vi "HTTPMethod_Synchronous_Simple.vi"(0 "LabVIEWHTTPClient_NET in":refnum<class "HttpClient_NET.lvclass">, 1 "input file":path, 2 "Method":T2, 3 "output file":path, 5 "URL":string, 7 "buffer":string, 9 "request headers":cluster{"header":string, "value":string}[](array[cluster]), 11 "error in (no error)":errorcluster, 12 "Timeout_ms (10000)":i32=10000) -> (4 "LabVIEWHTTPClient_NET out":refnum<class "HttpClient_NET.lvclass">, 6 "Headers":T1, 8 "Response":string, 10 "StatusCode":i32(ring)=100 items=["Continue"=100, "SwitchingProtocols"=101, "OK"=200, "Created"=201, "Accepted"=202, "NonAuthoritativeInformation"=203, "NoContent"=204, "ResetContent"=205, "PartialContent"=206, "MultipleChoices, Ambiguous"=300, "MovedPermanently, Moved"=301, "Found, Redirect"=302, "SeeOther, RedirectMethod"=303, "NotModified"=304, "UseProxy"=305, "Unused"=306, "TemporaryRedirect, RedirectKeepVerb"=307, "BadRequest"=400, "Unauthorized"=401, "PaymentRequired"=402, "Forbidden"=403, "NotFound"=404, "MethodNotAllowed"=405, "NotAcceptable"=406, "ProxyAuthenticationRequired"=407, "RequestTimeout"=408, "Conflict"=409, "Gone"=410, "LengthRequired"=411, "PreconditionFailed"=412, "RequestEntityTooLarge"=413, "RequestUriTooLong"=414, "UnsupportedMediaType"=415, "RequestedRangeNotSatisfiable"=416, "ExpectationFailed"=417, "UpgradeRequired"=426, "InternalServerError"=500, "NotImplemented"=501, "BadGateway"=502, "ServiceUnavailable"=503, "GatewayTimeout"=504, "HttpVersionNotSupported"=505], 13 "ReasonPhrase":string, 14 "Timeout":bool, 15 "error out":errorcluster)   [LabVIEW 2018, in "HttpClient_NET.lvlib" / "HttpClient_NET.lvclass"]
doc: "<b> </b> <b> </b>\nHttpClient_NET\nJustin Young - Viviota\nCopyright (c) 2021\nLicense: BSD"
uses:
  HttpClient_NET.lvclass
  Types/method_enum.ctl
  Types/ResponseHeaders_Cluster.ctl
  HttpHeaders_response/HttpHeaders_Response.lvclass
  HttpHeaders_content/HttpHeaders_Content.lvclass
  HttpResponseMessage/HttpResponseMessage.lvclass
  HttpRequestMessage/HttpRequestMessage.lvclass
  HttpClient_NET.lvlib
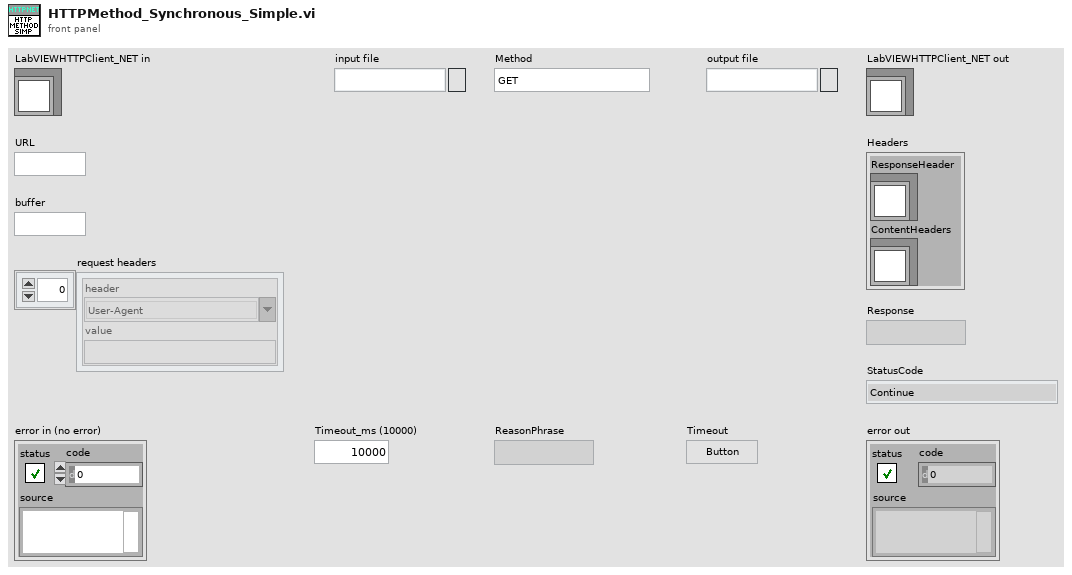
[diagram p1: front panel]
types:
  T1 = typedef "HttpClient_NET.lvlib/ResponseHeaders_Cluster.ctl" = cluster{"ResponseHeader":refnum<class "HttpHeaders_Response.lvclass">, "ContentHeaders":refnum<class "HttpHeaders_Content.lvclass">}
  T2 = typedef "HttpClient_NET.lvlib/method_enum.ctl" = enum16{"GET", "PUT", "POST", "DELETE", "HEAD", "TRACE", "SEND"}
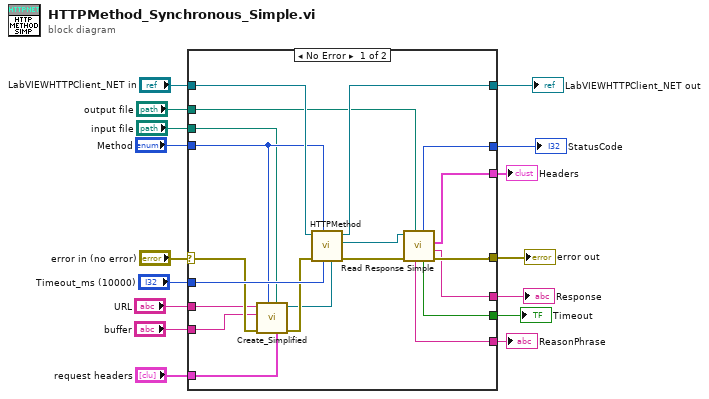
[diagram p0: block diagram]
diagram:
  n1 = case shown="No Error" "error in (no error)" {
    selector: "error in (no error)" -> [w25 w38]
    tunnel: [w32 w38] -> w15
    tunnel: [w34 w37] -> w13
    tunnel: "LabVIEWHTTPClient_NET in" -> [w35 w37]
    tunnel: "Method" -> [w22 _]
    tunnel: "Timeout_ms (10000)" -> [w36 _]
    tunnel: "URL" -> [w21 _]
    tunnel: "output file" -> [w30 _]
    tunnel: [w29 _] -> w8
    tunnel: [w28 _] -> w7
    tunnel: [w27 _] -> w3
    tunnel: [w26 _] -> w2
    tunnel: "input file" -> [w20 _]
    tunnel: "buffer" -> [w19 _]
    tunnel: "request headers" -> [w18 _]
    tunnel: [w17 _] -> w1
    frame No Error {
      n2 = call "Create_Simplified.vi"("request headers"=w18, "input file"=w20, "Method [GET]"=w22, "error in (no error)"=w25, "buffer"=w19, "Address"=w21) -> ("error out"=w24:errorcluster, "HttpRequestMessage out"=w23:refnum<class "HttpRequestMessage.lvclass">)  [unwired: 3 in, 1 out]
      n3 = call "HTTPMethod.vi"("HttpRequestMessage"=w23, "Timeout_ms (10000)"=w36, "Method"=w22, "error in (no error)"=w24, "LabVIEWHTTPClient_NET in"=w35) -> ("error out"=w33:errorcluster, "HttpResponseMessage out"=w31:refnum<class "HttpResponseMessage.lvclass">, "LabVIEWHTTPClient_NET out"=w34:refnum<class "HttpClient_NET.lvclass">)  [unwired: 4 in]
      n4 = call "Read Response Simple.vi"("output file"=w30, "error in (no error)"=w33, "HttpResponseMessage in"=w31) -> ("error out"=w32:errorcluster, "Response"=w28:string, "Headers"=w26:T1, "Timeout"=w29:bool, "StatusCode"=w27:i32, "ReasonPhrase"=w17:string)  [unwired: 3 in]
    }
    frame Error {
    }
  }
  "error out" <- w15
  "LabVIEWHTTPClient_NET out" <- w13
  "Timeout" <- w8
  "Response" <- w7
  "StatusCode" <- w3
  "Headers" <- w2
  "ReasonPhrase" <- w1
